vi "Fetch.vi"(8 "error in (no error)":errorcluster, 10 "Message in":refnum<class "FetchMessage.lvclass">, 11 "Chat in":refnum<class "Chat.lvclass">) -> (0 "error out":errorcluster, 3 "Chat out":refnum<class "Chat.lvclass">)   [LabVIEW 2012, in "Chat.lvclass"]
doc: "The fetch method processes the command 'fetch'. \n\nThe command 'fetch' is used for receiving various forms of data."
uses:
  Chat.lvclass
  <vilib>/Distrio/Murmex/FetchMessage/FetchMessage.lvclass
  <vilib>/Distrio/Murmex/Murmex/Murmex.lvclass
  <vilib>/Distrio/Murmex/Message/Message.lvclass
panel:
  # "This method is called when the FETCH\ntrigger is sent. \n\nOverride this method when your component needs to\nrespond to this trigger. \n\nCall parent for proper implementation"
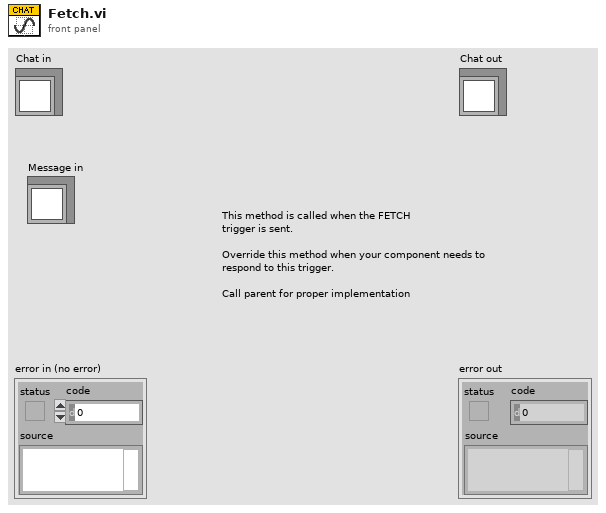
[diagram p1: front panel]
types:
  T1 = typedef "Murmex.lvlib/FetchMessage.lvclass/Channel data cluster.ctl" = cluster{"channel id":i32, "data UInt8":u8[], "data type":T2, "dimensions":i32[], "physical units":T3[], "waveform dt":dbl, "waveform":T4}
  T2 = typedef "Murmex.lvlib/Murmex.lvclass/data_type_enum.ctl" = enum16{"Float128", "Float64", "Float32", "Int64", "Int32", "Int16", "Int8", "UInt64", "UInt32", "UInt16", "UInt8", "Boolean", "String"}
  T3 = typedef "Murmex.lvlib/Murmex.lvclass/Physical Units.ctl" = cluster{"Base Units":enum16{"radian", "steradian", "second", "meter", "kilogram", "ampere", "kelvin", "mole", "candela"}, "Exponent":i16}
  T4 = typedef "Murmex.lvlib/Murmex.lvclass/waveform_type_enum.ctl" = enum16{"no waveform", "analog", "digital"}
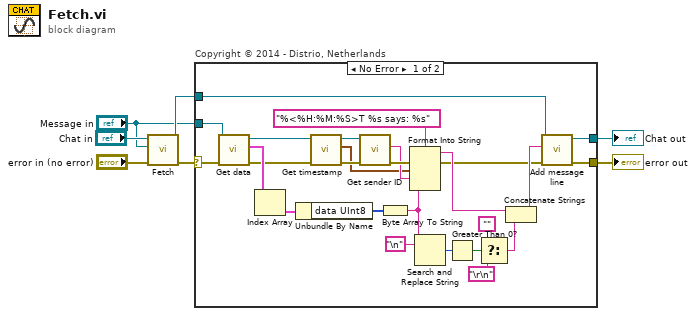
[diagram p0: block diagram]
diagram:
  n1 = call-parent "Fetch.vi"("error in (no error)"="error in (no error)", "Message in"="Message in", "Murmex in"="Chat in") -> ("error out"=w5:errorcluster, "Murmex out"=w4:refnum<class "Chat.lvclass">)  [unwired: 7 in]
  n2 = case "Copyright © 2014 - Distrio, Netherlands" shown="No Error" w5 {
    selector: w5 -> [w31 w35]
    tunnel: w4 -> [w29 w34]
    tunnel: "Message in" -> [w30 _]
    tunnel: [w33 w35] -> w2
    tunnel: [w32 w34] -> w1
    frame No Error {
      n3 = call <vilib>:"Get data.vi"("error in (no error)"=w31, "FetchMessage.lvclass"=w30) -> ("error out"=w19:errorcluster, "data (channels)"=w27:T1[], "FetchMessage out"=w20:refnum<class "FetchMessage.lvclass">)  [unwired: 7 in]
      n4 = Index Array(array=w27) -> (element=w28:T1)  [unwired: 1 in]
      n5 = Unbundle By Name(w28) -> ("data UInt8"=w26:u8[])
      n6 = call <vilib>:"Get timestamp.vi"("error in (no error)"=w19, "Message in"=w20) -> ("error out"=w18:errorcluster, "timestamp"=w17:timestamp, "Message out"=w21:refnum<class "FetchMessage.lvclass">)  [unwired: 7 in]
      n7 = call <vilib>:"Get sender ID.vi"("error in (no error)"=w18, "Message in"=w21) -> ("error out"=w25:errorcluster, "sender"=w24:string)  [unwired: 7 in, 1 out]
      n8 = Byte Array To String(unsigned byte array=w26) -> (string=w14:string)
      n9 = Format Into String(format string="%<%H:%M:%S>T %s says: %s", error in=w25, w17, w24, w14) -> (resulting string=w22:string, error out=w8:errorcluster)  [unwired: 1 in]
      n10 = Search and Replace String(input string=w14, search string="\n") -> (number of replacements=w16:i32)  [unwired: 6 in, 3 out]
      n11 = Greater Than 0?(x=w16) -> (x > 0?=w13:bool)
      n12 = Select(t="", s=w13, f="\r\n") -> (s? t:f=w12:string)
      n13 = Concatenate Strings(w22, w12) -> (w9:string)
      n14 = call "Add message line.vi"("error in (no error)"=w8, "Message in"=w9, "Chat in"=w29) -> ("error out"=w33:errorcluster, "Chat out"=w32:refnum<class "Chat.lvclass">)  [unwired: 7 in]
    }
    frame Error {
    }
  }
  "error out" <- w2
  "Chat out" <- w1
